vi "close.vi"(8 "errorIn":errorcluster, 11 "refer":refnum<queue>) -> (0 "errorOut":errorcluster)   [LabVIEW 2017]
uses:
  models/EMSGData.ctl
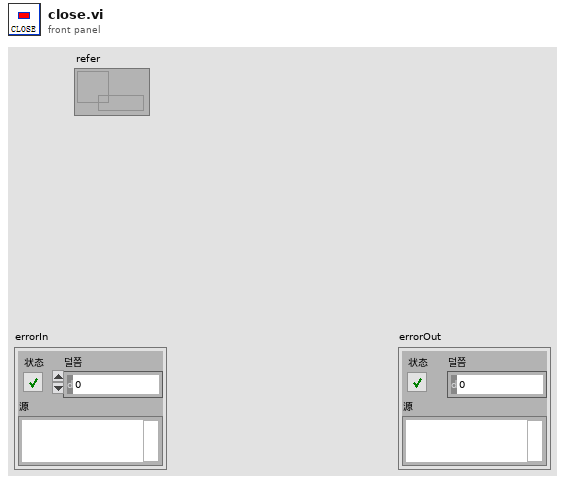
[diagram p1: front panel]
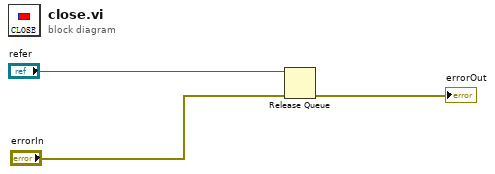
[diagram p0: block diagram]
diagram:
  n1 = Release Queue(queue="refer", error in (no error)="errorIn") -> (error out=→"errorOut":errorcluster)  [unwired: 1 in, 2 out]
